vi "Cmd.HandlePositiveResponse.vi"(1 "Response":string) -> (0 "ResponseParameters":string[](array[string]))   [LabVIEW 2016]
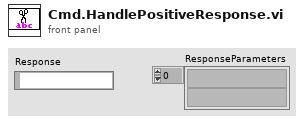
[diagram p1: front panel]
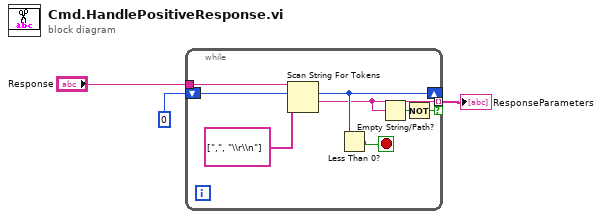
[diagram p0: block diagram]
diagram:
  n1 = while {
    tunnel: "Response" -> [w11]
    tunnel: [w6] -> w3 mode=indexing if=w4
    shift-right: [w8] -> _
    shift-left: 0 -> [w10]
    stop <- w7 stop-if-true
    n2 = Scan String For Tokens(6:string[] [",", "\\r\\n"], 8:w10, 9:w11) -> (1:w6:string, 2:w8:i32)  [unwired: 3 in, 2 out]
    n3 = Less Than 0?(x=w8) -> (x < 0?=w7:bool)
    n4 = Empty String/Path?(string/path=w6) -> (empty?=w5:bool)
    n5 = Not(x=w5) -> (.not. x?=w4:bool)
  }
  "ResponseParameters" <- w3
